vi "PROG 4 - String Practice.vi"() -> ()   [LabVIEW 2012]
panel:
  in  "Combo Box":string(combo)
  out "String 2":string
  in  "String":string
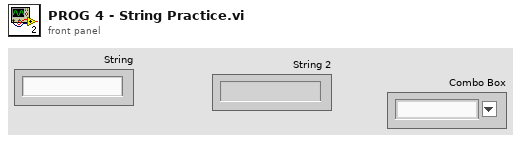
[diagram p1: front panel]
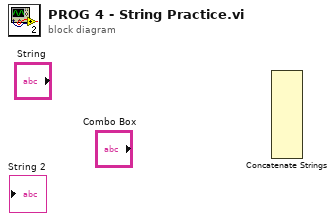
[diagram p0: block diagram]
diagram:
  n1 = Concatenate Strings() -> ()  [unwired: 11 in, 1 out]
